vi "Get Last Temperature.vi"(8 "error in":errorcluster, 10 "Channel":string, 11 "Thermometer DAQmx RTD Cont CFG in":refnum<class "Thermometer DAQmx RTD Cont CFG.lvclass">) -> (0 "error out":errorcluster, 2 "Temperature":dbl, 3 "Thermometer DAQmx RTD Cont CFG out":refnum<class "Thermometer DAQmx RTD Cont CFG.lvclass">)   [LabVIEW 2024, in "Thermometer DAQmx RTD Cont CFG.lvclass"]
uses:
  Thermometer DAQmx RTD Cont CFG.lvclass
  Thermometer DAQmx RTD Cont CFG.lvclass/Thermometer DAQmx RTD Cont CFG.ctl
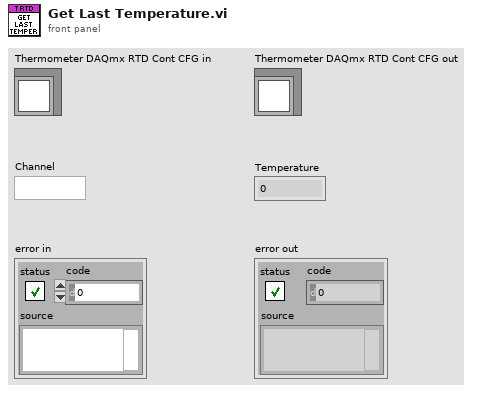
[diagram p1: front panel]
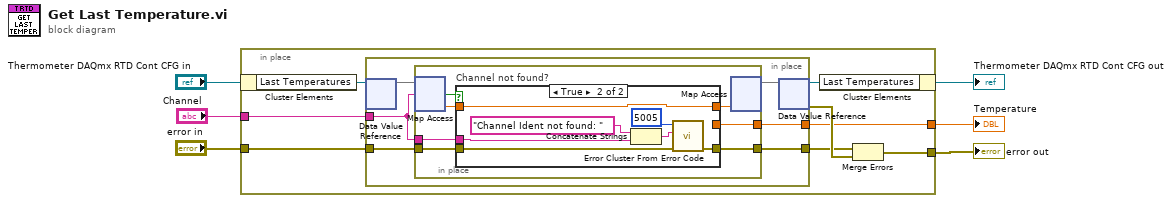
[diagram p0: block diagram]
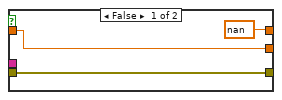
[diagram p2: hidden frame]
diagram:
  n1 = in-place {
    in-place-border: "Channel" -> [w13]
    in-place-border: "error in" -> [w12]
    in-place-border: [w10] -> w5
    in-place-border: [w8] -> w1
    n2 = in-place-cluster #1("Thermometer DAQmx RTD Cont CFG in") -> ("Last Temperatures"=w14:refnum<data-value>)
    n3 = in-place {
      in-place-border: w13 -> [w17]
      in-place-border: w12 -> [w19]
      in-place-border: [w18] -> w8
      in-place-border: [w16] -> w7
      n4 = in-place-dvr #2(w14) -> (w20:map{string, dbl})  [unwired: 1 out]
      n5 = in-place {
        in-place-border: w19 -> [w26]
        in-place-border: [w24] -> w18
        in-place-border: w17 -> [w22]
        in-place-border: [w21] -> w16
        n6 = in-place-map #3(w20, w17) -> (w25:dbl, w27:bool)  [unwired: 1 in]
        n7 = case "Channel not found?" shown="True" w27 {
          tunnel: [w28 w34] -> w21
          tunnel: w26 -> [w28 w33]
          tunnel: w25 -> [w30 w31]
          tunnel: [w30 _] -> w24
          tunnel: [nan w31] -> w23
          tunnel: w22 -> [_ w32]
          frame False {
          }
          frame True {
            n8 = Concatenate Strings("Channel Ident not found: " ("error message (\"\")"), w32) -> (w36:string)
            n9 = call <vilib>:"Error Cluster From Error Code.vi"("error in (no error)"=w33, "error message (\"\")"=w36, "error code (0)"=5005) -> ("error out"=w34:errorcluster)  [unwired: 6 in]
          }
        }
        n10 = in-place-map #3(w23) -> (w15:map{string, dbl})  [unwired: 1 in, 2 out]
      }
      n11 = in-place-dvr #2(w15) -> (w11:refnum<data-value>, w9:errorcluster)
    }
    n12 = in-place-cluster #1("Last Temperatures"=w11) -> (→"Thermometer DAQmx RTD Cont CFG out":refnum<class "Thermometer DAQmx RTD Cont CFG.lvclass">)
    n13 = Merge Errors(w7, w9) -> (w10:errorcluster)
  }
  "error out" <- w5
  "Temperature" <- w1
